vi "ViewPicts.vi"(0 "Choose Directory":path) -> ()   [LabVIEW 2022 SP3]
panel:
  in  "Smooth factor":i32=3
  in  "lower dB limit":dbl=-50.0
  in  "Use Selected Files":bool
  in  "Listbox":i32[](listbox)
  in  "Columns":i32=3
  in  "reduce RF pts by factor of":i32=10
  in  "pixels in y":i16=160
  in  "pixels in x":i16=200
  out "Array":picture[][](array[picture])
  # "© 2000 Riverside Research Institute"
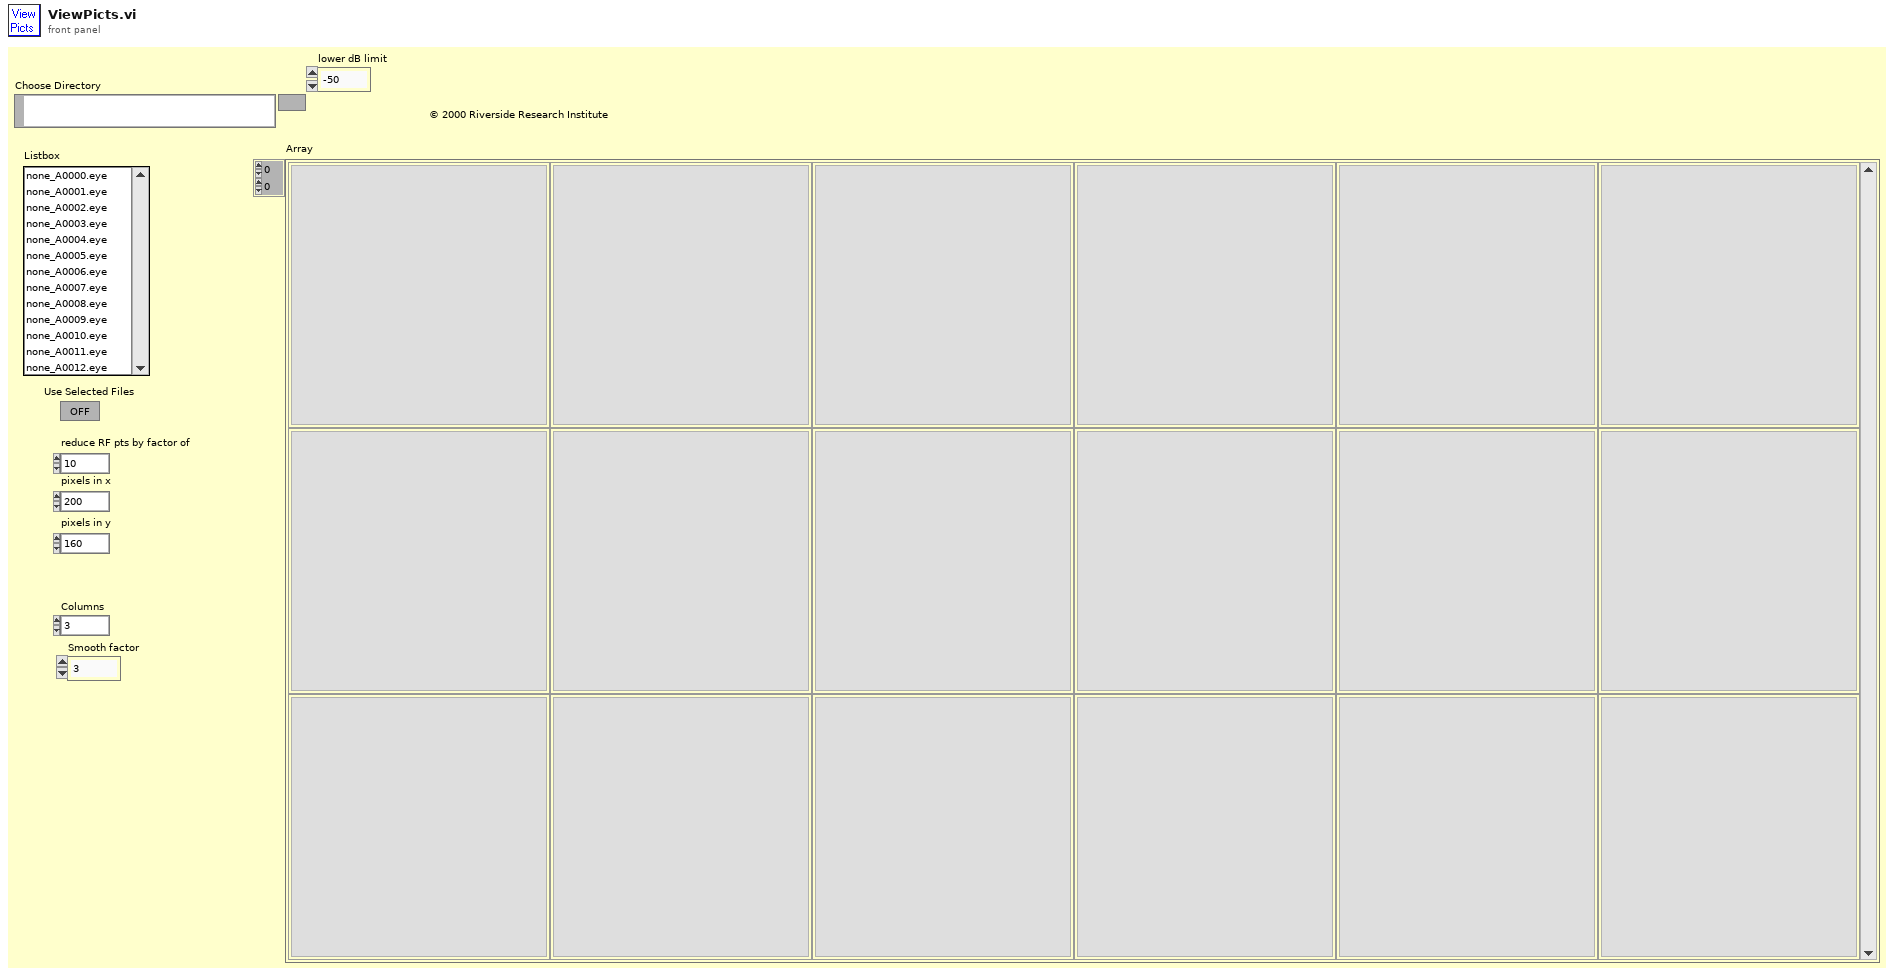
[diagram p1: front panel]
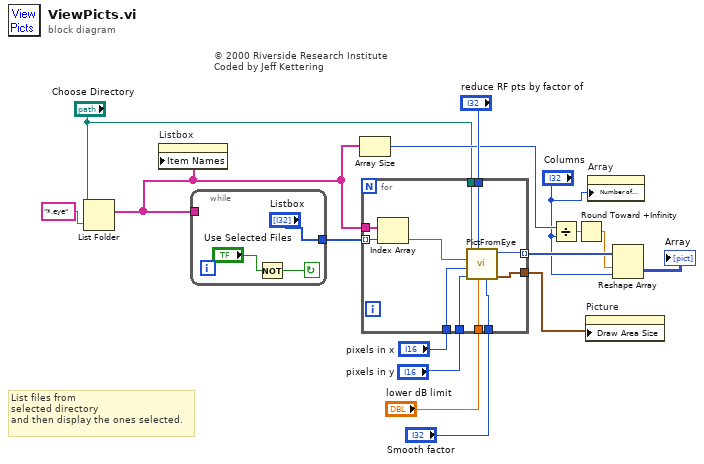
[diagram p0: block diagram]
diagram:
  # "© 2000 Riverside Research Institute\nCoded by Jeff Kettering"
  # "List files from\nselected directory\nand then display the ones selected."
  n1 = List Folder(path="Choose Directory", pattern="*.eye") -> (filenames=w7:string[])  [unwired: 1 in, 4 out]
  n2 = property on="Listbox" class="LstBox (strict)"("Item Names"=w7) -> ()  [unwired: 2 in, 2 out]
  n3 = while {
    tunnel: w7 -> [_]
    tunnel: ["Listbox"] -> w8
    stop <- w18 continue-if-true
    n4 = Not(x="Use Selected Files") -> (.not. x?=w18:bool)
  }
  n5 = Array Size(array=w7) -> (size(s)=w6:i32)
  n6 = for {
    tunnel: "pixels in x" -> [w30]
    tunnel: "pixels in y" -> [w29]
    tunnel: "Choose Directory" -> [w28]
    tunnel: [w27] -> w13 mode=indexing
    tunnel: [w26] -> w12
    tunnel: "reduce RF pts by factor of" -> [w25]
    tunnel: w8 -> [w24] mode=indexing
    tunnel: w7 -> [w23]
    tunnel: "lower dB limit" -> [w21]
    tunnel: "Smooth factor" -> [w20]
    n7 = Index Array(array=w23, index=w24) -> (element=w22:string)
    n8 = call "PictFromEye.vi"("Smooth factor"=w20, "lower dB limit"=w21, "reduce pts by factor of"=w25, "pixels in y"=w29, "pixels in x"=w30, "file name"=w22, "file path directory"=w28) -> ("Picture Size"=w26:cluster{"pixels in x":i16, u16}, "Sector as picture"=w27:picture)  [unwired: 3 in]
  }
  n9 = Divide(x=w6, y="Columns") -> (x/y=w10:dbl)
  n10 = Round Toward +Infinity(x=w10) -> (ceil(x): smallest int >= x=w5:dbl)
  n11 = property on="Picture" class="Pict"("Draw Area Size"=w12) -> ()  [unwired: 2 in, 2 out]
  n12 = property on="Array" class="Arr (strict)"("Number of Columns"="Columns") -> ()  [unwired: 2 in, 2 out]
  n13 = Reshape Array(w13, w5, "Columns") -> (→"Array":picture[][])
